vi "My.SMO.UI.SetConfiguration.vi"(8 "error in (no error)":errorcluster, 10 "Configuration":T1, 11 "My.SMO.UI":refnum<class "My.SMO.UI.lvclass">) -> (0 "error out":errorcluster, 3 "My.SMO.UI out":refnum<class "My.SMO.UI.lvclass">)   [LabVIEW 2016, in "My.SMO.UI.lvclass"]
doc: "---------------------------------------------------------------\nJKI State Machine Objects™\nhttp://jki.net/state-machine-objects/\nCopyright (C) 2005-2015, JKI <info@jki.net>\nALL RIGHTS RESERVEDJKI State Machine Objects (SMO) 1.0.0.5\nJKI - JKI\nCopyright (c) 2016, JKI"
uses:
  My.SMO.UI.lvclass
  Typedefs/Configuration--Cluster.ctl
  My.SMO.UI.lvclass/My.SMO.UI.ctl
panel:
  # "For instructions on how to use the JKI State Machine Objects, examples and video tutorials, visit:\nhttp://jki.net/state-machine-objects/\n\nJKI State Machine Objects™\nhttp://jki.net/state-machine-objects/\nCopyright (C) 2005-2015, JKI <info@jki.net>\nALL RIGHTS RESERVED"
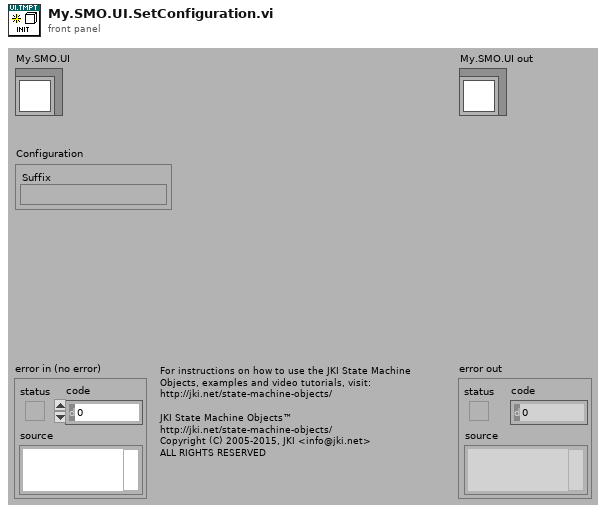
[diagram p1: front panel]
types:
  T1 = typedef "My.SMO.UI.lvclass/Configuration--Cluster.ctl" = cluster{"Suffix":string}
  T2 = typedef "My.SMO.UI.lvclass/PrivateData--Ref.ctl" = refnum<data-value>
  T3 = typedef "My.SMO.UI.lvclass/PrivateData--Cluster.ctl" = cluster{"Configuration":T1, "Public Events":T4, "Protected Events":T5, "Data":string}
  T4 = typedef "My.SMO.UI.lvclass/PublicEvents--Cluster.ctl" = cluster{"Data Changed":refnum<user-event>}
  T5 = typedef "My.SMO.UI.lvclass/ProtectedEvents--Cluster.ctl" = cluster{"API_Template":refnum<user-event>}
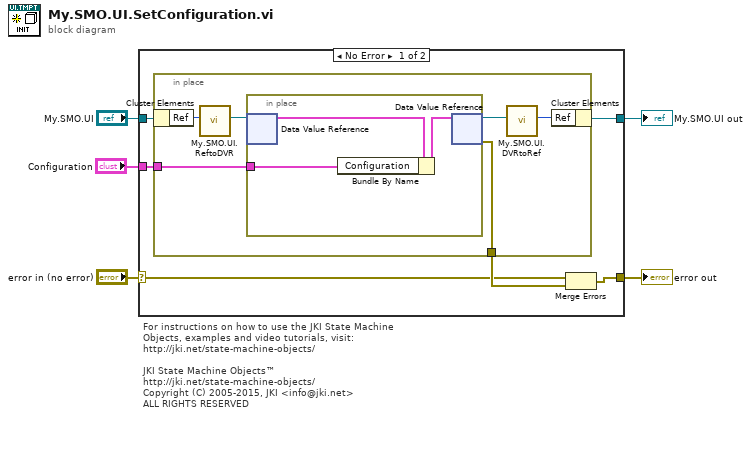
[diagram p0: block diagram]
diagram:
  # "For instructions on how to use the JKI State Machine Objects, examples and video tutorials, visit:\nhttp://jki.net/state-machine-objects/\n\nJKI State Machine Objects™\nhttp://jki.net/state-machine-objects/\nCopyright (C) 2005-2015, JKI <info@jki.net>\nALL RIGHTS RESERVED"
  n1 = case shown="No Error" "error in (no error)" {
    selector: "error in (no error)" -> [w6 w21]
    tunnel: "My.SMO.UI" -> [w7 w22]
    tunnel: [w8 w21] -> w4
    tunnel: [w11 w22] -> w3
    tunnel: "Configuration" -> [w10 _]
    frame No Error {
      n2 = in-place {
        in-place-border: w10 -> [w17]
        in-place-border: [w16] -> w9
        n3 = in-place-cluster #1(w7) -> ("Ref"=w15:u32)
        n4 = call "My.SMO.UI.ReftoDVR.vi"("Ref"=w15) -> ("Ref"=w14:T2)  [unwired: 10 in]
        n5 = in-place {
          in-place-border: w17 -> [w18]
          n6 = in-place-dvr #2(w14) -> (w20:T3)  [unwired: 1 out]
          n7 = Bundle By Name(cluster=w20, "Configuration"=w18) -> (w19:T3)
          n8 = in-place-dvr #2(w19) -> (w13:T2, w16:errorcluster)
        }
        n9 = call "My.SMO.UI.DVRtoRef.vi"("Ref"=w13) -> ("Ref"=w12:u32)  [unwired: 10 in]
        n10 = in-place-cluster #1("Ref"=w12) -> (w11:refnum<class "My.SMO.UI.lvclass">)
      }
      n11 = Merge Errors(w6, w9) -> (w8:errorcluster)
    }
    frame Error {
    }
  }
  "error out" <- w4
  "My.SMO.UI out" <- w3
